vi "Close Leds and Dut Selectors.vi"(7 "SWD Sel Task":refnum<k21>, 8 "error in":errorcluster, 9 "RF Switch Sel Task":refnum<k21>, 10 "Dut2 Leds Task":refnum<k21>, 11 "Dut1 Leds Task":refnum<k21>) -> (0 "error out":errorcluster)   [LabVIEW 2018]
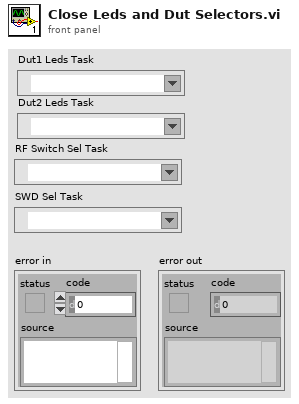
[diagram p1: front panel]
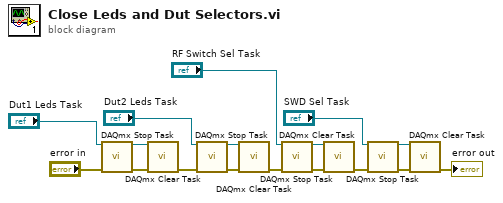
[diagram p0: block diagram]
diagram:
  n1 = call <vilib>:"DAQmx Stop Task.vi"("task/channels in"="Dut1 Leds Task", "error in"="error in") -> ("task out"=w13:refnum<k21>, "error out"=w12:errorcluster)  [unwired: 12 in]
  n2 = call <vilib>:"DAQmx Clear Task.vi"("task in"=w13, "error in"=w12) -> ("error out"=w9:errorcluster)  [unwired: 13 in]
  n3 = call <vilib>:"DAQmx Stop Task.vi"("task/channels in"="Dut2 Leds Task", "error in"=w9) -> ("task out"=w17:refnum<k21>, "error out"=w16:errorcluster)  [unwired: 12 in]
  n4 = call <vilib>:"DAQmx Clear Task.vi"("task in"=w17, "error in"=w16) -> ("error out"=w6:errorcluster)  [unwired: 13 in]
  n5 = call <vilib>:"DAQmx Stop Task.vi"("task/channels in"="RF Switch Sel Task", "error in"=w6) -> ("task out"=w15:refnum<k21>, "error out"=w14:errorcluster)  [unwired: 12 in]
  n6 = call <vilib>:"DAQmx Clear Task.vi"("task in"=w15, "error in"=w14) -> ("error out"=w2:errorcluster)  [unwired: 13 in]
  n7 = call <vilib>:"DAQmx Stop Task.vi"("task/channels in"="SWD Sel Task", "error in"=w2) -> ("task out"=w5:refnum<k21>, "error out"=w3:errorcluster)  [unwired: 12 in]
  n8 = call <vilib>:"DAQmx Clear Task.vi"("task in"=w5, "error in"=w3) -> ("error out"=→"error out":errorcluster)  [unwired: 13 in]
